vi "DisplayConsole_ModuleCommunicationQueue.vi"(5 "Who send this":T1, 7 "Action":T2, 8 "error in (no error)":errorcluster, 10 "ModuleData":variant) -> (0 "error out":errorcluster, 3 "Ref out":refnum<queue>, 4 "# elements in queue":i32)   [LabVIEW 2013]
doc: "This is Display Console module communication queue. You can communicate with this module using this queue. \n\nThis is Functional Global Variable."
uses:
  General/Controls/#TD_General_FromWho_Enum.ctl
  General/Controls/#TD_General_IntermoduleData_Cluster.ctl
  General/Controls/#TD_General_CommunicationQueueStates_Enum.ctl
panel:
  # "INPUT"
  # "OUTPUT"
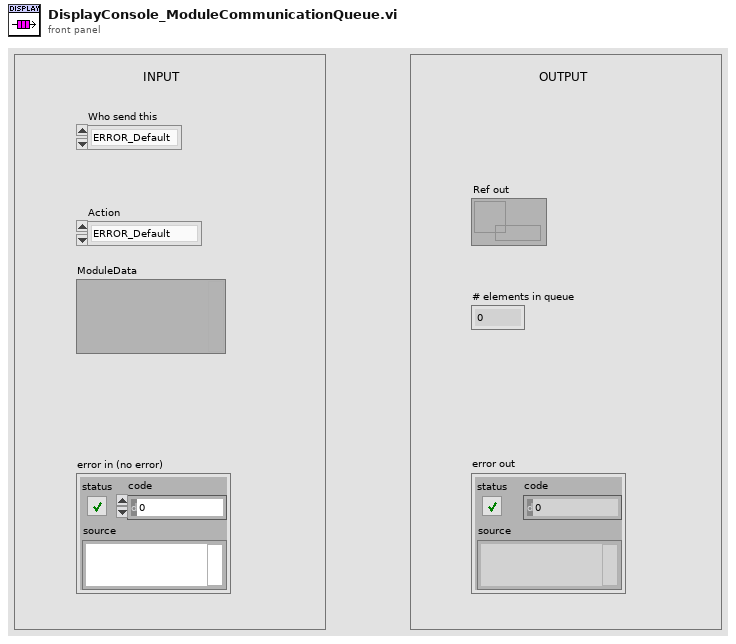
[diagram p1: front panel]
types:
  T1 = typedef "#TD_General_FromWho_Enum.ctl" = enum16{"ERROR_Default", "UserConsole", "DisplayConsole", "SensorInterface", "Controller", "Database", "Timing", "ErrorHandling"}
  T2 = typedef "#TD_General_CommunicationQueueStates_Enum.ctl" = enum16{"ERROR_Default", "Obtain", "GetRef", "Enqueue", "EnqueueAtOpp", "GetStatus", "Release"}
  T3 = typedef "#TD_General_IntermoduleData_Cluster.ctl" = cluster{"Sender":T1, "ModuleData":variant}
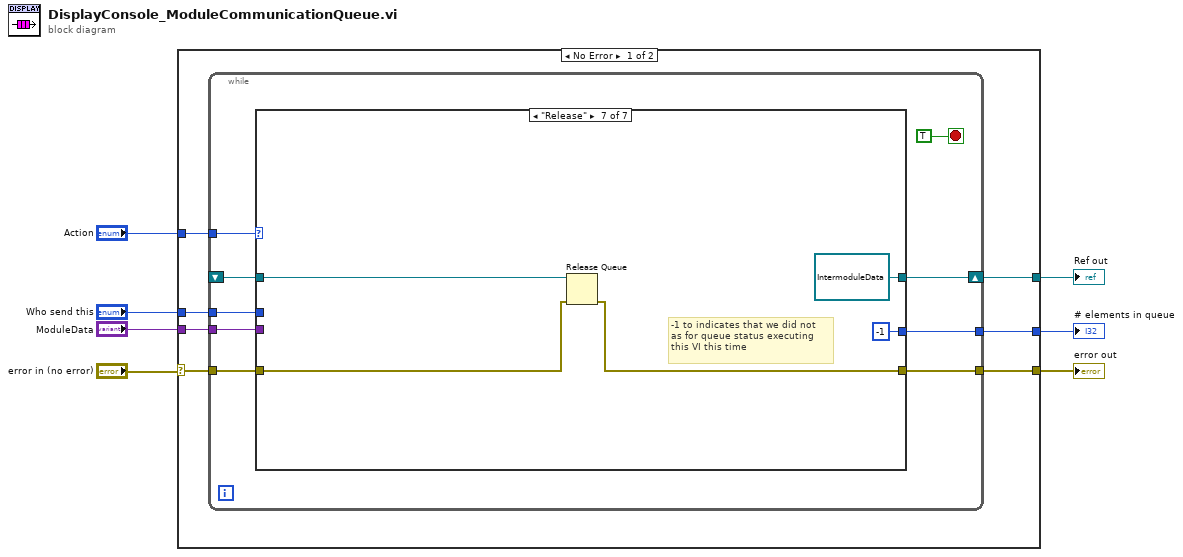
[diagram p0: block diagram]
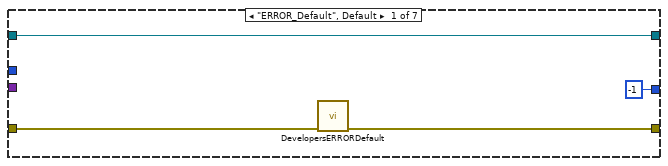
[diagram p2: hidden frame]
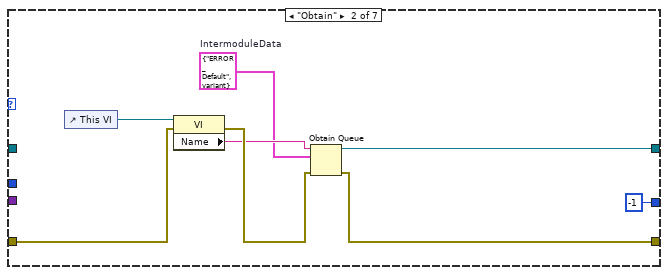
[diagram p3: hidden frame]
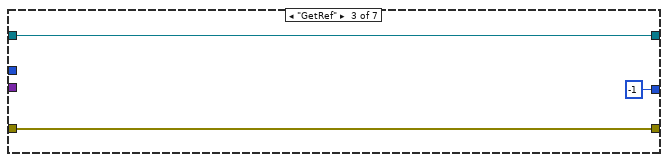
[diagram p4: hidden frame]
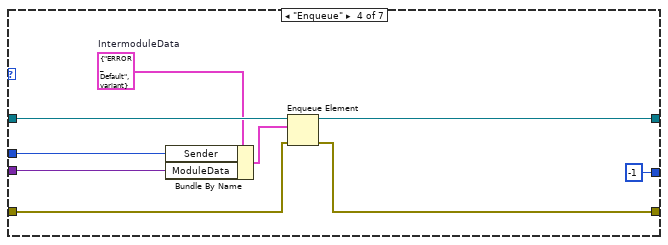
[diagram p5: hidden frame]
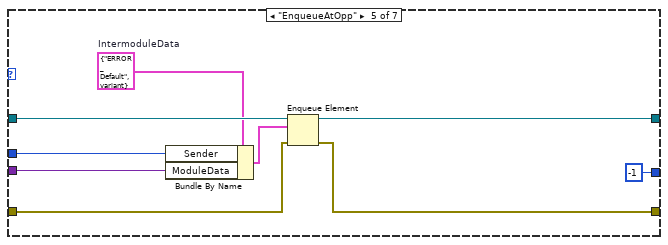
[diagram p6: hidden frame]
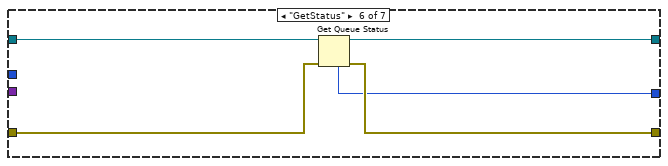
[diagram p7: hidden frame]
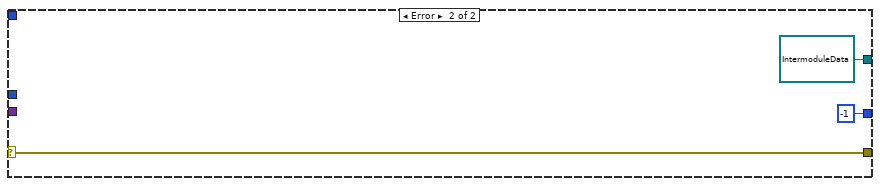
[diagram p8: hidden frame]
diagram:
  n1 = case shown="No Error" "error in (no error)" {
    selector: "error in (no error)" -> [w13 w69]
    tunnel: "Action" -> [w14 _]
    tunnel: [w12 w69] -> w5
    tunnel: [w11 refnum<queue> refnum ("queue out")] -> w4
    tunnel: "Who send this" -> [w10 _]
    tunnel: "ModuleData" -> [w9 _]
    tunnel: [w8 -1 ("# elements in queue")] -> w1
    frame No Error {
      n2 = while {
        tunnel: w14 -> [w22]
        tunnel: w13 -> [w21]
        tunnel: [w20] -> w12
        shift-right: [w19] -> w11
        shift-left: _ -> [w18]
        tunnel: w10 -> [w17]
        tunnel: w9 -> [w16]
        tunnel: [w15] -> w8
        stop <- TRUE stop-if-true
        n3 = case shown="\"Release\"" w22 {
          tunnel: w21 -> [w27 w33 w37 w44 w53 w61 w65]
          tunnel: [w26 w35 w37 w45 w54 w60 w64] -> w20
          tunnel: [w24 w30 w38 w46 w55 w58 refnum<queue> refnum ("queue out")] -> w19
          tunnel: w18 -> [w24 _ w38 w47 w56 w59 w66]
          tunnel: w17 -> [_ _ _ w41 w50 _ _]
          tunnel: w16 -> [_ _ _ w40 w49 _ _]
          tunnel: [-1 ("# elements in queue") -1 ("# elements in queue") -1 ("# elements in queue") -1 ("# elements in queue") -1 ("# elements in queue") w57 -1 ("# elements in queue")] -> w15
          frame "ERROR_Default", Default {
            n4 = call "DevelopersERRORDefault.vi"("error in (no error)"=w27) -> ("error out"=w26:errorcluster)  [unwired: 10 in]
          }
          frame "Obtain" {
            w29 = T3 {"Sender"=enum."ERROR_Default", "ModuleData"=variant}  # IntermoduleData
            n5 = control-ref of="This VI"() -> (w34:refnum<vi>)
            n6 = property class="VI"(reference=w34, error in=w33) -> (error out=w32:errorcluster, "Name"=w31:string)  [unwired: 1 out]
            n7 = Obtain Queue(name (unnamed)=w31, element data type=w29, error in (no error)=w32) -> (queue out=w30:refnum<queue>, error out=w35:errorcluster)  [unwired: 2 in, 1 out]
          }
          frame "GetRef" {
          }
          frame "Enqueue" {
            w43 = T3 {"Sender"=enum."ERROR_Default", "ModuleData"=variant}  # IntermoduleData
            n8 = Bundle By Name(cluster=w43, "Sender"=w41, "ModuleData"=w40) -> (w42:T3)
            n9 = Enqueue Element(queue=w47, element=w42, error in (no error)=w44) -> (queue out=w46:refnum<queue>, error out=w45:errorcluster)  [unwired: 1 in, 1 out]
          }
          frame "EnqueueAtOpp" {
            w52 = T3 {"Sender"=enum."ERROR_Default", "ModuleData"=variant}  # IntermoduleData
            n10 = Bundle By Name(cluster=w52, "Sender"=w50, "ModuleData"=w49) -> (w51:T3)
            n11 = Enqueue Element(queue=w56, element=w51, error in (no error)=w53) -> (queue out=w55:refnum<queue>, error out=w54:errorcluster)  [unwired: 1 in, 1 out]
          }
          frame "GetStatus" {
            n12 = Get Queue Status(queue=w59, error in (no error)=w61) -> (queue out=w58:refnum<queue>, error out=w60:errorcluster, # elements in queue=w57:i32)  [unwired: 1 in, 5 out]
          }
          frame "Release" {
            # "-1 to indicates that we did not \nas for queue status executing \nthis VI this time"
            n13 = Release Queue(queue=w66, error in (no error)=w65) -> (error out=w64:errorcluster)  [unwired: 1 in, 2 out]
          }
        }
      }
    }
    frame Error {
    }
  }
  "error out" <- w5
  "Ref out" <- w4
  "# elements in queue" <- w1
